vi "Test_WriteString_NoFormatString_WriteExactString.vi"(8 "error in (no error)":errorcluster, 11 "TestCase in":refnum<class "TestFormattedStringBinding.lvclass">) -> (0 "error out":errorcluster, 3 "TestCase out":refnum<class "TestFormattedStringBinding.lvclass">)   [LabVIEW 2017, in "TestFormattedStringBinding.lvclass"]
uses:
  TestFormattedStringBinding.lvclass
  Source/Concrete/FormattedStringBinding/FormattedStringBinding.lvclass/FormattedStringBinding.ctl
  Source/Concrete/FormattedStringBinding/FormattedStringBinding.lvclass
  C:/Git/composed-transport/Source/Concrete/TerminalValueBinding/TerminalValueBinding.lvclass
  C:/Git/composed-transport/Source/ITransport/ITransport.lvclass
  <vilib>/Utility/error.llb/Error Cluster From Error Code.vi
  Source/Concrete/TerminalValueBinding/Construct Terminal Value Binding.vi
  Source/ITransport/ITransport.lvclass
panel:
  in  "String":string
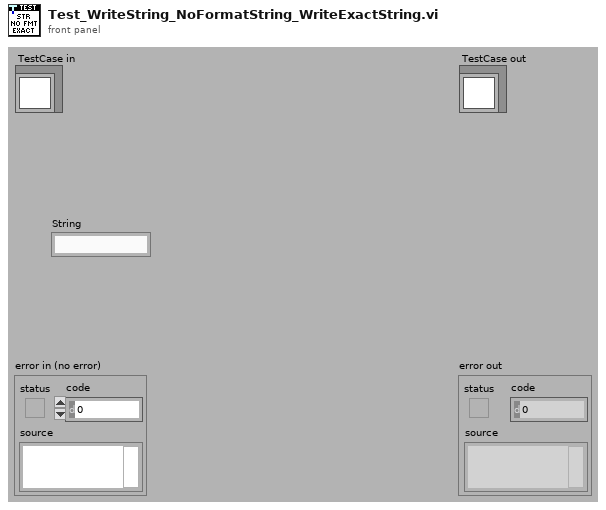
[diagram p1: front panel]
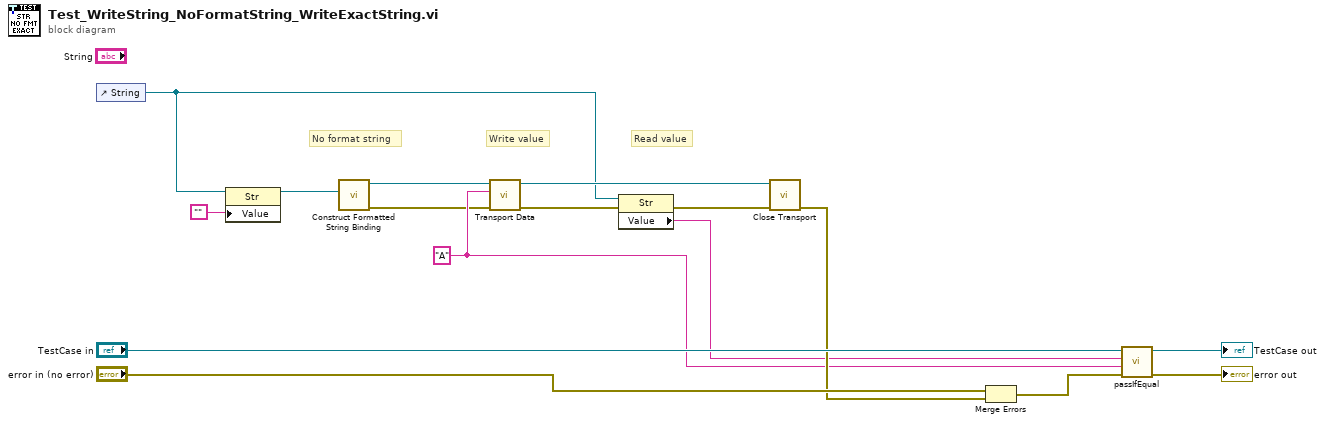
[diagram p0: block diagram]
diagram:
  w3 = "A" ("Format String")
  # "Read value"
  # "No format string"
  # "Write value"
  n1 = control-ref of="String"() -> (w2:refnum<vi>)
  n2 = property class="Str"(reference=w2, "Value"="") -> (reference out=w8:refnum<vi>)  [unwired: 1 in, 1 out]
  n3 = call "Construct Formatted String Binding.vi"("Str Refnum"=w8) -> ("error out"=w1:errorcluster, "FormattedStringBinding"=w12:refnum<class "FormattedStringBinding.lvclass">)  [unwired: 9 in]
  n4 = call "Transport Data.vi"("error in (no error)"=w1, "Value"=w3, "ITransport in"=w12) -> ("error out"=w6:errorcluster, "ITransport out"=w10:refnum<class "FormattedStringBinding.lvclass">)  [unwired: 7 in]
  n5 = property class="Str"(reference=w2, error in=w6) -> (error out=w5:errorcluster, "Value"=w4:string)  [unwired: 1 out]
  n6 = call-dynamic "Close Transport.vi"("error in (no error)"=w5, "ITransport in"=w10) -> ("error out"=w9:errorcluster)  [unwired: 9 in]
  n7 = Merge Errors("error in (no error)", w9) -> (w11:errorcluster)
  n8 = call-dynamic "passIfEqual.vi"("error in (no error)"=w11, "y"=w3, "x"=w4, "TestCase in"="TestCase in") -> ("error out"=→"error out":errorcluster, "TestCase out"=→"TestCase out":refnum<class "TestFormattedStringBinding.lvclass">)  [unwired: 6 in]
